vi "NOT a CSM.vi"   [LabVIEW 2017]
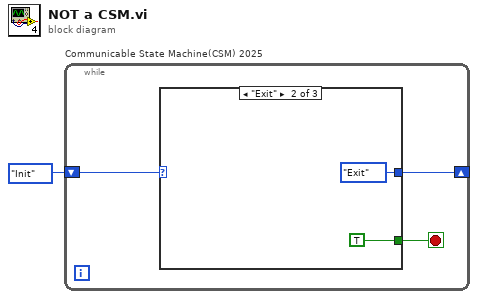
[diagram p0: block diagram]
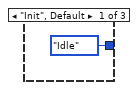
[diagram p2: hidden frame]
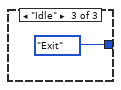
[diagram p3: hidden frame]
diagram:
  n1 = while "Communicable State Machine(CSM) 2025" {
    shift-right: [w3] -> _
    shift-left: enum16{"Init", "Idle", "Exit"}."Init" -> [w4]
    stop <- w2 stop-if-true
    n2 = case shown="\"Exit\"" w4 {
      tunnel: [enum16{"Init", "Idle", "Exit"}."Idle" enum16{"Init", "Idle", "Exit"}."Exit" enum16{"Init", "Idle", "Exit"}."Exit"] -> w3
      tunnel: [_ TRUE _] -> w2
      frame "Init", Default {
      }
      frame "Exit" {
      }
      frame "Idle" {
      }
    }
  }
